vi "Launcher.vi"() -> ()   [LabVIEW 2019, in "Project Build Tools.lvclass"]
uses:
  Project Build Tools.lvclass
  TypeDefs/Configure Build Types.ctl
  Project Build Tools.lvclass/Project Build Tools.ctl
panel:
  in  "Project Path":path
  out "Errors":errorcluster
  out "Build Progress":u8(slide) scale=0.0..100.0
  out "Current Build":string
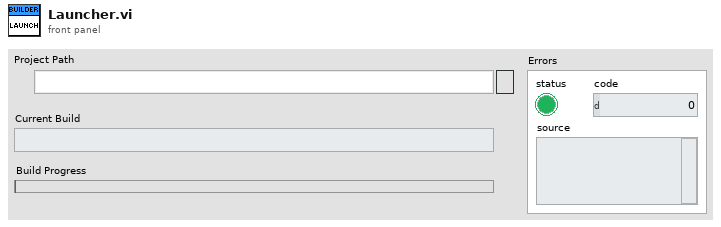
[diagram p1: front panel]
types:
  T1 = typedef "Project Build Tools.lvclass/Configure Build Types.ctl" = enum16{"DLL", "Packed Library", "Installer", "Source Distribution", "EXE"}
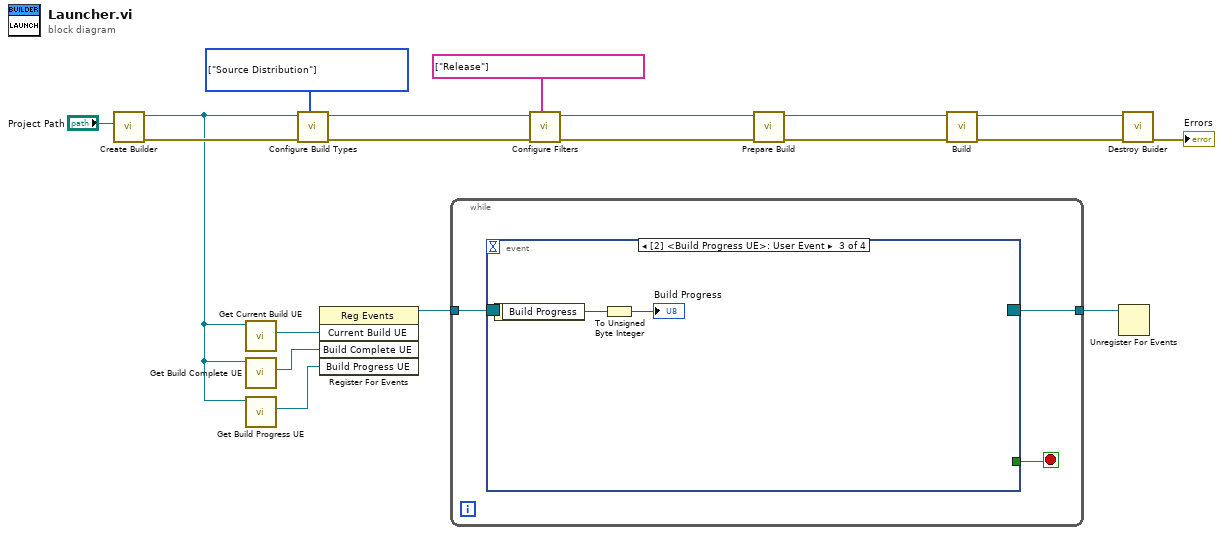
[diagram p0: block diagram]
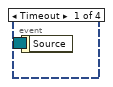
[diagram p2: hidden frame]
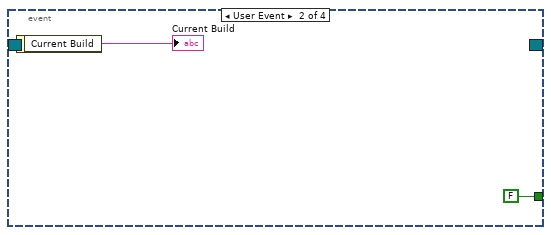
[diagram p3: hidden frame]
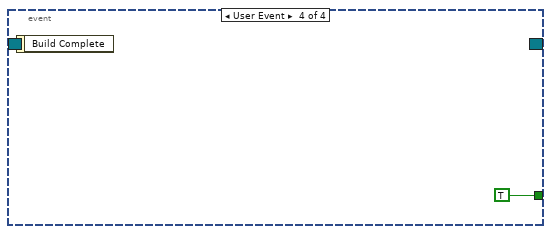
[diagram p4: hidden frame]
diagram:
  w1 = T1[] [enum."Source Distribution"] items=["DLL", "Packed Library", "Installer", "Source Distribution", "EXE"] ("Build Types")
  n1 = call "Create Builder.vi"("File Path Control"="Project Path") -> ("error out"=w6:errorcluster, "CD Build Tools out"=w5:refnum<class "Project Build Tools.lvclass">)  [unwired: 9 in]
  n2 = call "Get Current Build UE.vi"("CD Build Tools in"=w5) -> ("Current Build UE"=w10:refnum<user-event>)  [unwired: 9 in, 1 out]
  n3 = call "Get Build Complete UE.vi"("CD Build Tools in"=w5) -> ("Build Complete UE"=w8:refnum<user-event>)  [unwired: 9 in, 1 out]
  n4 = call "Get Build Progress UE.vi"("CD Build Tools in"=w5) -> ("Build Progress UE"=w4:refnum<user-event>)  [unwired: 9 in, 1 out]
  n5 = call "Configure Build Types.vi"("Build Types"=w1, "error in (no error)"=w6, "CD Build Tools in"=w5) -> ("error out"=w19:errorcluster, "CD Build Tools out"=w18:refnum<class "Project Build Tools.lvclass">)  [unwired: 7 in]
  n6 = register-events(w10, w8, w4) -> (reference out=w9:refnum<event-registration>)  [unwired: 2 in, 1 out]
  n7 = while {
    tunnel: w9 -> [w22]
    tunnel: [w20] -> w7
    stop <- w21 stop-if-true
    n8 = event shown="[2] <Build Progress UE>: User Event" {
      selector: w22 -> [_ _ _ _]
      dyn-events: [_ _ _ _] -> w20
      timeout: _ -> [_ _ _ _]
      tunnel: [_ FALSE _ TRUE] -> w21
      event Timeout {
        n9 = event-data() -> ()  [unwired: 1 in, 1 out]
      }
      event User Event {
        n10 = event-data() -> ("Current Build"=→"Current Build":string)  [unwired: 1 in]
      }
      event User Event {
        n11 = event-data() -> ("Build Progress"=w26:i32)  [unwired: 1 in]
        n12 = To Unsigned Byte Integer(number=w26) -> (unsigned 8bit integer=→"Build Progress":u8)
      }
      event User Event {
        n13 = event-data() -> ()  [unwired: 1 in, 1 out]
      }
    }
  }
  n14 = call "Configure Filters.vi"("Name Filters"=string[] ["Release"] ("Filters"), "error in (no error)"=w19, "CD Build Tools in"=w18) -> ("error out"=w17:errorcluster, "CD Build Tools out"=w16:refnum<class "Project Build Tools.lvclass">)  [unwired: 7 in]
  n15 = call "Prepare Build.vi"("error in (no error)"=w17, "CD Build Tools in"=w16) -> ("error out"=w11:errorcluster, "CD Build Tools out"=w12:refnum<class "Project Build Tools.lvclass">)  [unwired: 8 in]
  n16 = call "Build.vi"("error in (no error)"=w11, "CD Build Tools in"=w12) -> ("error out"=w13:errorcluster, "CD Build Tools out"=w14:refnum<class "Project Build Tools.lvclass">)  [unwired: 7 in, 1 out]
  n17 = Unregister For Events(event registration refnum=w7) -> ()  [unwired: 1 in, 1 out]
  n18 = call "Destroy Buider.vi"("error in (no error)"=w13, "CD Build Tools in"=w14) -> ("error out"=→"Errors":errorcluster)  [unwired: 9 in]
